vi "Ctor Device.vi"(8 "error in (no error)":errorcluster, 11 "Simulated Waveform in":refnum<class "Simulated Waveform.lvclass">) -> (0 "error out":errorcluster, 3 "Simulated Waveform out":refnum<class "Simulated Waveform.lvclass">)   [LabVIEW 2020, in "Simulated Waveform.lvlib" / "Simulated Waveform.lvclass"]
uses:
  Simulated Waveform.lvclass
  Ref Data.ctl
  Simulated Waveform.lvclass/Simulated Waveform.ctl
  build/ppl/Signal Generator.lvlibp/Signal Generator/Signal Generator.lvclass
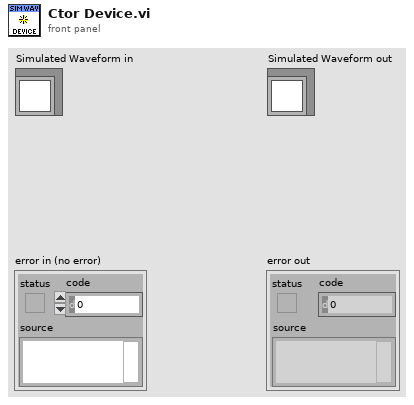
[diagram p1: front panel]
types:
  T1 = typedef "Simulated Waveform.lvlib/Simulated Waveform.lvclass/Ref Data.ctl" = cluster{"Sim Queue Name":string, "Waveform Queue":refnum<queue>, "Noise Factor":dbl}
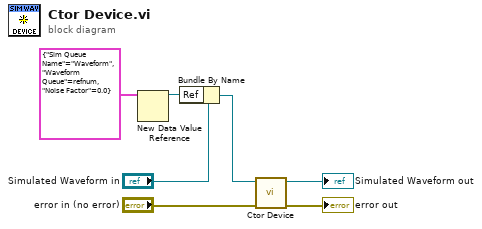
[diagram p0: block diagram]
diagram:
  n1 = New Data Value Reference(data value=T1 {"Sim Queue Name"="Waveform", "Waveform Queue"=refnum, "Noise Factor"=0.0} ("Ref Data")) -> (data value reference=w5:refnum<data-value>)  [unwired: 1 in, 1 out]
  n2 = Bundle By Name(cluster="Simulated Waveform in", "Ref"=w5) -> (w3:refnum<class "Simulated Waveform.lvclass">)
  n3 = call-parent "Ctor Device.vi"("error in (no error)"="error in (no error)", "Signal Generator in"=w3) -> ("error out"=→"error out":errorcluster, "Signal Generator out"=→"Simulated Waveform out":refnum<class "Simulated Waveform.lvclass">)  [unwired: 8 in]
